vi "4.3.vi"() -> ()   [LabVIEW 2017]
panel:
  out "平均值":dbl
  in  "数值":dbl
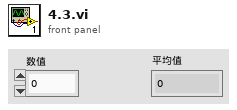
[diagram p1: front panel]
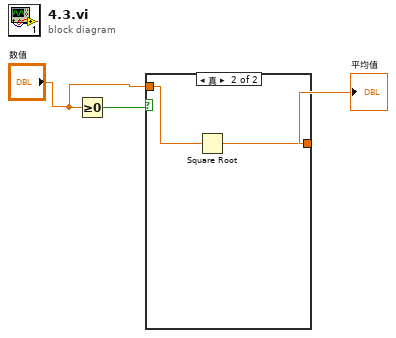
[diagram p0: block diagram]
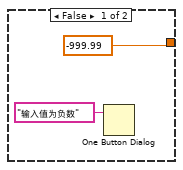
[diagram p2: hidden frame]
diagram:
  n1 = Greater Or Equal To 0?(x="数值") -> (x >= 0?=w2:bool)
  n2 = case shown="真" w2 {
    tunnel: [-999.99 w7] -> w3
    tunnel: "数值" -> [_ w6]
    frame False {
      n3 = One Button Dialog(message="输入值为负数" ("消息")) -> ()  [unwired: 1 in, 1 out]
    }
    frame True {
      n4 = Square Root(x=w6) -> (sqrt(x)=w7:dbl)
    }
  }
  "平均值" <- w3
